vi "Generate Sound_chirp.vi"(0 "Device ID":u32, 1 "Start Frequency":dbl=500.0, 5 "chirp duration [s]":dbl=-1.0, 9 "amplitude":dbl=1.0 format="%.2f", 11 "sampling info":cluster{"Fs":dbl, "#s":u32}={"Fs"=51200.0, "#s"=1024} {"Fs" format="%.2p"}, 12 "Stop":bool, 13 "Stop Frequency":dbl=500.0) -> ()   [LabVIEW 2021]
doc: "This VI illustrates how to generate and play sine, square, sawtooth and triangle waveforms. You can change the frequency and type of the waveform generated as it plays continuously."
uses:
  <vilib>/sound2/lvsound2.llb/Sampling Mode.ctl
  <vilib>/sound2/lvsound2.llb/Sound Data Format.ctl
  <vilib>/sound2/lvsound2.llb/Sound Output Set Volume (Single).vi
  <vilib>/sound2/lvsound2.llb/Sound Output Write (DBL Single).vi
  <vilib>/addons/_NISVFA/_Generation/SoundVib_Generation.lvlib
panel:
  in  "Volume":dbl(slide)=50.0 scale=0.0..100.0
  # "Overview: Demonstrates the use of the Sound Functions to generate and play a sine waveform continuously.\nInstructions:\n1. Specify the Device ID.\n2. Run the VI. Waveforms are generated and sent to both the graph and your speakers.\n3. Change the Frequency and Volume of the sound.\n4. Click Stop to stop the VI."
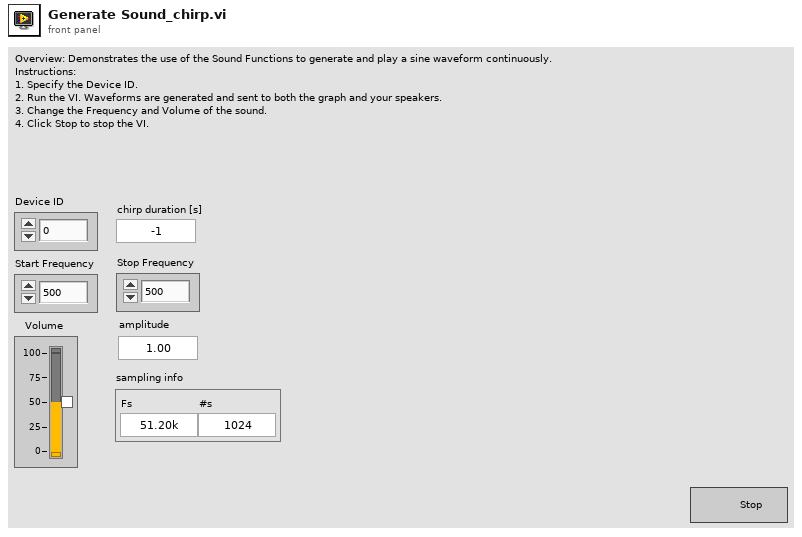
[diagram p1: front panel]
types:
  T1 = typedef "Sound Data Format.ctl" = cluster{"sample rate (S/s)":dbl, "number of channels":i32, "bits per sample":i32}
  T2 = typedef "Sampling Mode.ctl" = i32
  T3 = typedef "Sound Output Task ID.ctl" = u32
  T4 = cluster{"start frequency [Hz]":dbl, "stop frequency [Hz]":dbl}
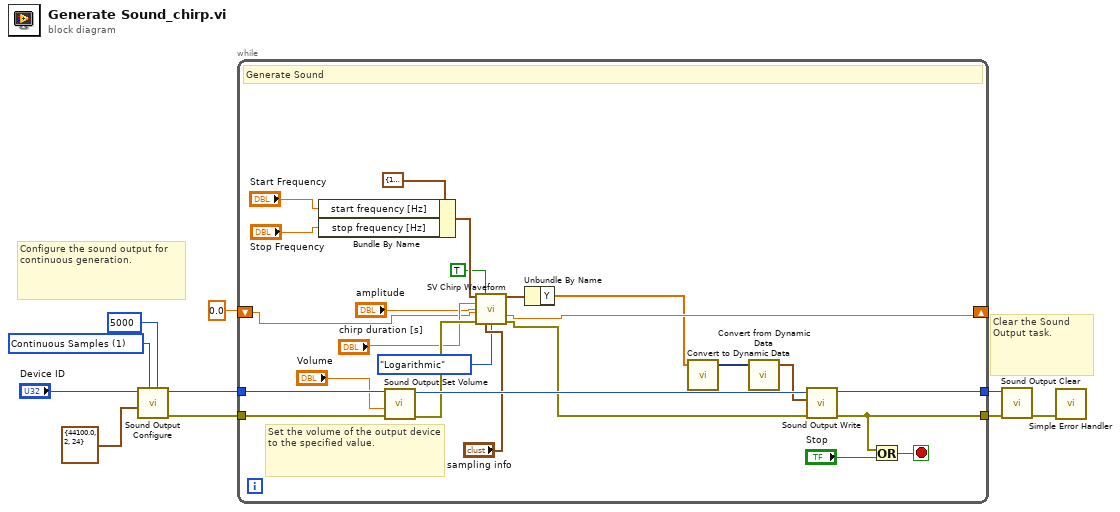
[diagram p0: block diagram]
diagram:
  w5 = T2 1 items=["Finite Samples", "Continuous Samples"] ("sample mode")
  # "Configure the sound output for continuous generation."
  # "Clear the Sound Output task."
  n1 = call <vilib>:"Sound Output Configure.vi"("number of samples/ch"=5000 ("Number of Samples/ch"), "sample mode"=w5, "sound format"=T1 {"sample rate (S/s)"=44100.0, "number of channels"=2, "bits per sample"=24} ("Sound Format"), "device ID"="Device ID") -> ("error out"=w10:errorcluster, "task ID"=w9:T3)  [unwired: 6 in]
  n2 = while {
    tunnel: w9 -> [w30]
    tunnel: [w35] -> w7
    tunnel: w10 -> [w32]
    tunnel: [w28] -> w8
    shift-right: [w19] -> _
    shift-left: 0.0 -> [w20]
    stop <- w33 stop-if-true
    # "Set the volume of the output device to the specified value."
    # "Generate Sound"
    n3 = Bundle By Name(cluster=T4 {"start frequency [Hz]"=10.0, "stop frequency [Hz]"=10000.0} ("frequency range"), "start frequency [Hz]"="Start Frequency", "stop frequency [Hz]"="Stop Frequency") -> (w23:T4)
    n4 = call-poly <vilib>:"Sound Output Set Volume.vi"("error in (no error)"=w32, "volume"="Volume", "task ID"=w30) -> ("error out"=w26:errorcluster, "task ID out"=w31:T3)  [unwired: 7 in]
    n5 = call <vilib>:"SV Chirp Waveform.vi"("frequency range"=w23, "reset signal (F)"=TRUE, "chirp duration [s]"="chirp duration [s]", "amplitude"="amplitude", "phase in [deg]"=w20, "error in (no error)"=w26, "sampling info"="sampling info", "frequency spacing"=enum16{"Linear", "Logarithmic"}."Logarithmic") -> ("chirp signal"=w16:waveform(dbl), "phase out [deg]"=w19:dbl, "error out"=w17:errorcluster)  [unwired: 5 in]
    n6 = Unbundle By Name(w16) -> ("Y"=w14:dbl[])
    n7 = call "Convert to Dynamic Data"("Array"=w14) -> ("Dynamic Data Type"=w15:dynamicdata)  [unwired: 3 in]
    n8 = call "Convert from Dynamic Data"("Dynamic Data Type"=w15) -> ("Waveform"=w12:waveform(dbl))  [unwired: 3 in]
    n9 = call-poly <vilib>:"Sound Output Write.vi"("error in (no error)"=w17, "data"=w12, "task ID"=w31) -> ("error out"=w28:errorcluster, "task ID out"=w35:T3)  [unwired: 7 in]
    n10 = Or(x=w28, y="Stop") -> (x .or. y?=w33:bool)
  }
  n11 = call <vilib>:"Sound Output Clear.vi"("error in (no error)"=w8, "task ID"=w7) -> ("error out"=w3:errorcluster)  [unwired: 9 in]
  n12 = call <vilib>:"Simple Error Handler.vi"("error in (no error)"=w3) -> ()  [unwired: 4 in, 5 out]
